vi "quiz 3.3.vi"() -> ()   [LabVIEW 2017]
panel:
  out "output string":string
  out "array":string[][](array[string])
  out "Tab Control":T1(tab)
  in  "Ingresar":bool
  in  "usuario":string
  in  "Contraseña":string
  in  "eliminar":bool
  in  "agregar":bool
  in  "TERMINAR":bool
  in  "Volver":bool
  in  "añadir":bool
  in  "contraseña":string
  in  "usuario":string
  in  "Quitar":bool
  in  "usuario a eliminar":string
  out "Seccion Inicada por:":string
  # "¿QUE DESEA REALIZAR?"
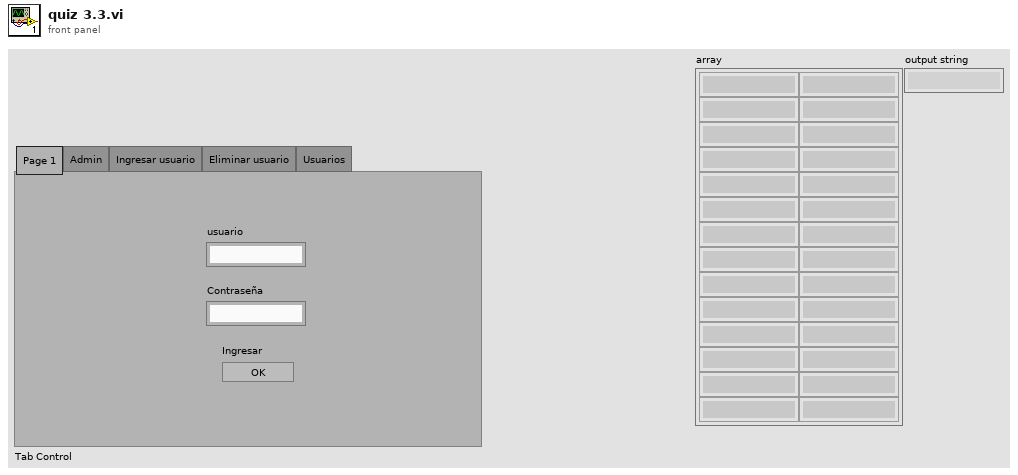
[diagram p1: front panel]
types:
  T1 = enum32{"Page 1", "Admin", "Ingresar usuario", "Eliminar usuario", "Usuarios"}
  T2 = enum16{"open", "replace", "create", "open or create", "replace or create", "replace or create with confirmation"}
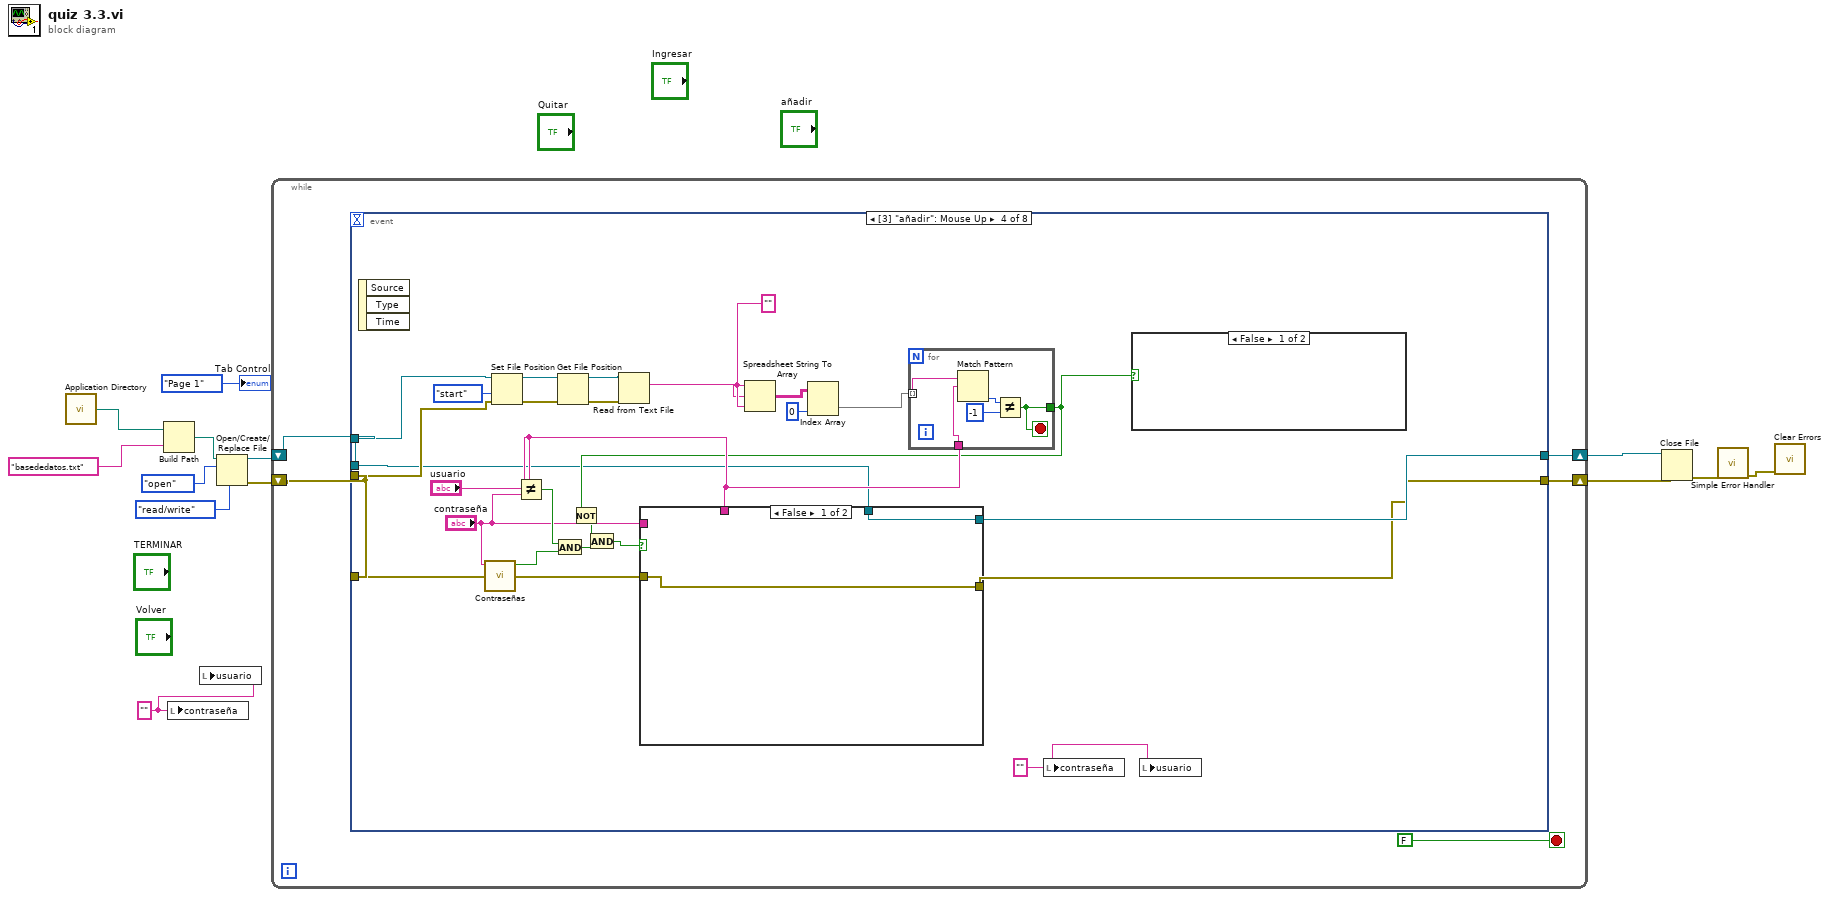
[diagram p0: block diagram]
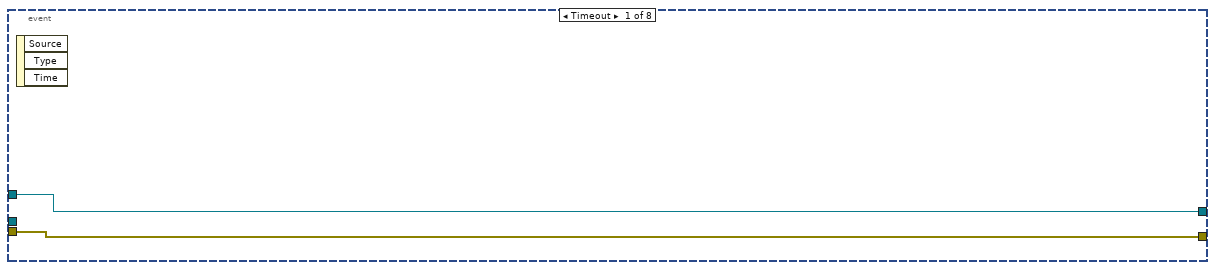
[diagram p2: hidden frame]
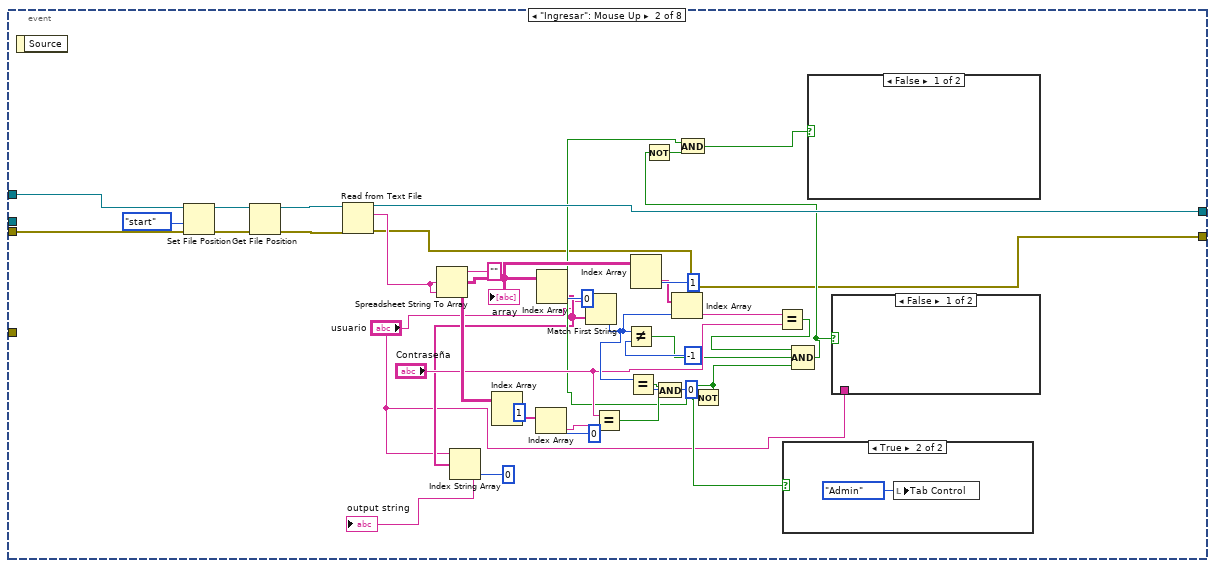
[diagram p3: hidden frame]
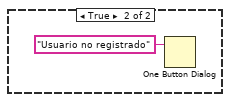
[diagram p4: hidden frame]
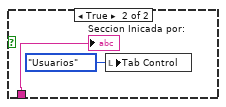
[diagram p5: hidden frame]
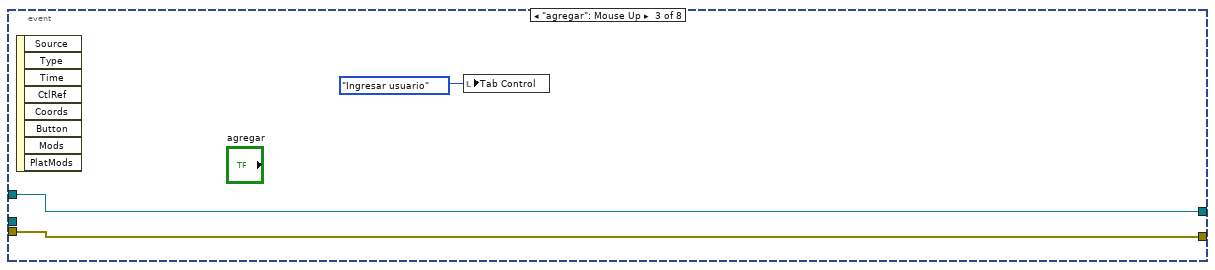
[diagram p7: hidden frame]
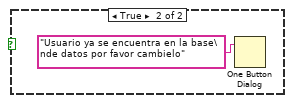
[diagram p8: hidden frame]
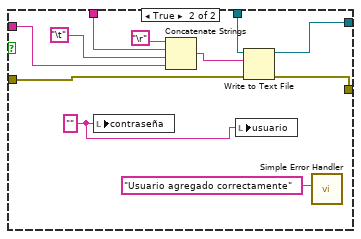
[diagram p9: hidden frame]
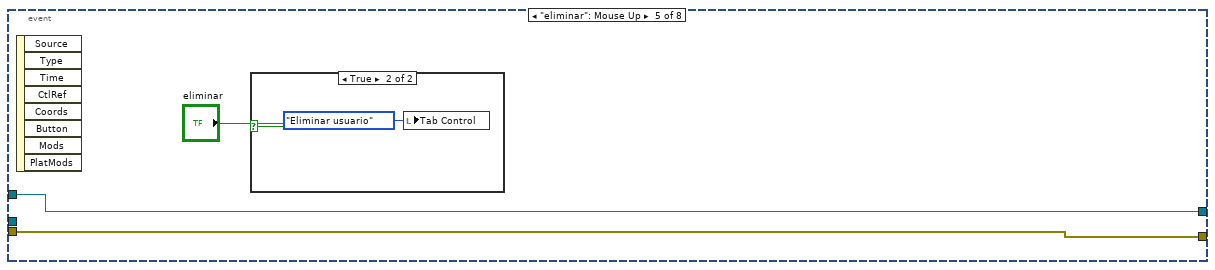
[diagram p10: hidden frame]
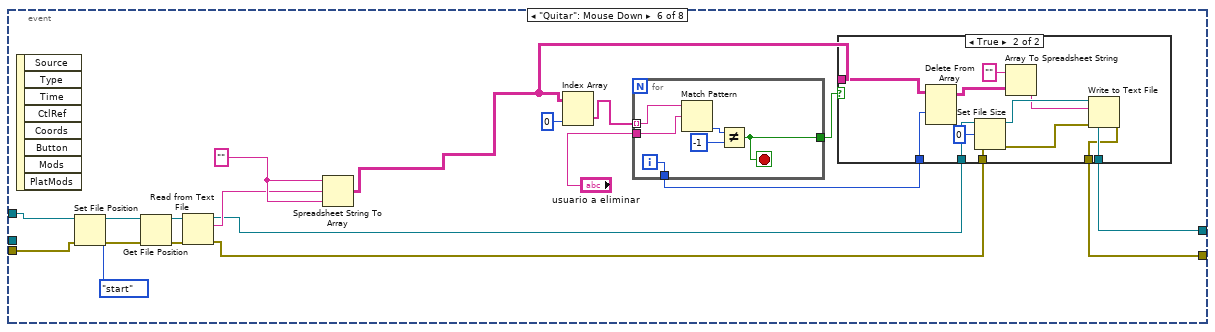
[diagram p12: hidden frame]
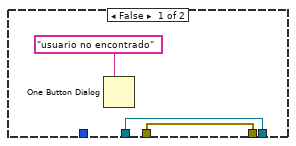
[diagram p13: hidden frame]
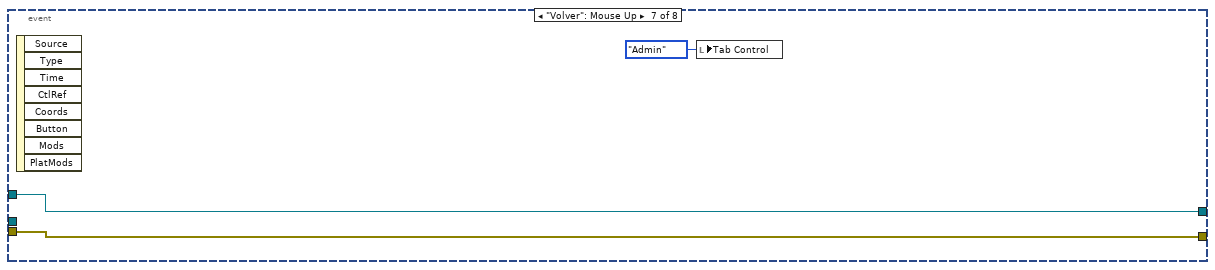
[diagram p14: hidden frame]
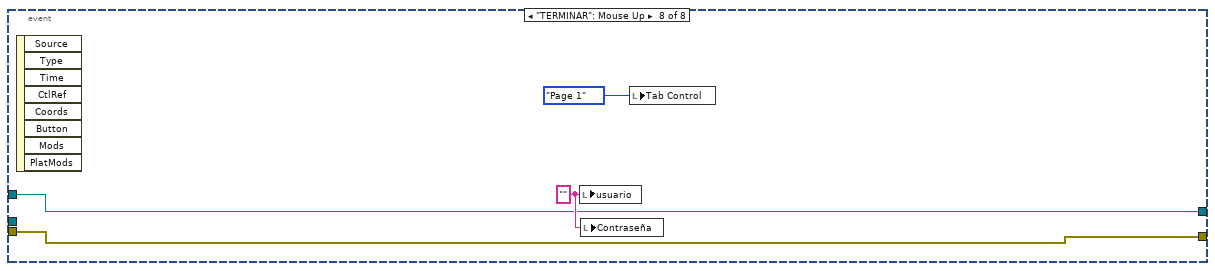
[diagram p15: hidden frame]
diagram:
  w1 = "" ("contraseña")
  n1 = call <vilib>:"Application Directory.vi"() -> ("Application Directory"=w10:path)
  n2 = Build Path(base path=w10, name or relative path="basededatos.txt") -> (appended path=w7:path)
  n3 = local write "contraseña"(w1) -> ()
  n4 = local write "usuario"(w1) -> ()
  n5 = Open/Create/Replace File(file path (use dialog)=w7, operation (0:open)=T2."open", access (0:read/write)=enum16{"read/write", "read-only", "write-only"}."read/write") -> (refnum out=w8:refnum<file>, error out=w5:errorcluster)  [unwired: 3 in, 1 out]
  n6 = while {
    shift-right: [w15] -> w11
    shift-left: w8 -> [w14]
    shift-right: [w16] -> w6
    shift-left: w5 -> [w17]
    stop <- FALSE stop-if-true
    n7 = event shown="[3] \"añadir\": Mouse Up" {
      selector: _ -> [_ _ _ _ _ _ _ _]
      dyn-events: _ -> [_ _ _ _ _ _ _ _]
      timeout: _ -> [_ _ _ _ _ _ _ _]
      tunnel: w14 -> [w20 w53 w64 w67 w109 w121 w154 w157]
      tunnel: [w20 w52 w64 w86 w109 w114 w154 w157] -> w15
      tunnel: w17 -> [w19 w48 w62 w82 w110 w120 w153 w156]
      tunnel: w17 -> [_ _ _ w88 _ _ _ _]
      tunnel: [w19 w22 w62 w69 w110 w113 w153 w156] -> w16
      tunnel: w14 -> [_ _ _ w66 _ _ _ _]
      event Timeout {
        n8 = event-data() -> ()  [unwired: 1 in, 3 out]
      }
      event "Ingresar": Mouse Up {
        n9 = event-data() -> ()  [unwired: 1 in, 1 out]
        n10 = Set File Position(refnum=w53, from (0:start)=enum16{"start", "end", "current"}."start", error in=w48) -> (refnum out=w57:refnum<file>, error out=w55:errorcluster)  [unwired: 1 in]
        n11 = Get File Position(4:w55, 7:w57) -> (0:w54:errorcluster, 3:w56:refnum<file>)  [unwired: 1 out]
        n12 = Read from Text File(file (use dialog)=w56, error in=w54) -> (refnum out=w52:refnum<file>, text=w50:string, error out=w22:errorcluster)  [unwired: 2 in, 1 out]
        n13 = Spreadsheet String To Array(format string="", spreadsheet string=w50, array type (2D Dbl)=w50) -> (array=w37:string[][])  [unwired: 1 in]
        "array" <- w37
        n14 = Index Array(array=w37, index (col)=1 ("disabled index (col)")) -> (element=w42:string[])  [unwired: 1 in]
        n15 = Index Array(array=w42, index=0) -> (element=w40:string)
        n16 = Index Array(array=w37, index (col)=0 ("disabled index (col)")) -> (element=w25:string[])  [unwired: 1 in]
        n17 = Index String Array(1:0 ("index"), 2:w25, 3:"usuario") -> (0:→"output string":string)
        n18 = Match First String(2:w25, 3:"usuario") -> (0:w34:i32)  [unwired: 1 out]
        n19 = Equal?(x="Contraseña", y=w40) -> (x = y?=w39:bool)
        n20 = Not Equal?(x=w34, y=-1) -> (x != y?=w30:bool)
        n21 = Equal?(x=w34, y=0) -> (x = y?=w44:bool)
        n22 = Index Array(array=w37, index (col)=1 ("disabled index (col)")) -> (element=w35:string[])  [unwired: 1 in]
        n23 = And(x=w44, y=w39) -> (x .and. y?=w38:bool)
        n24 = Index Array(array=w35, index=w34) -> (element=w33:string)
        n25 = Not(x=w38) -> (.not. x?=w26:bool)
        n26 = Equal?(x=w33, y="Contraseña") -> (x = y?=w31:bool)
        n27 = case shown="True" w38 {
          frame False {
          }
          frame True {
            n28 = local write "Tab Control"(T1."Admin" ("Tab Control")) -> ()
          }
        }
        n29 = Compound Arithmetic op=AND(w31, w30, w26) -> (w28:bool)
        n30 = Not(x=w28) -> (.not. x?=w29:bool)
        n31 = And(x=w26, y=w29) -> (x .and. y?=w27:bool)
        n32 = case shown="False" w27 {
          frame False {
          }
          frame True {
            n33 = One Button Dialog(message="Usuario no registrado") -> ()  [unwired: 1 in, 1 out]
          }
        }
        n34 = case shown="False" w28 {
          tunnel: "usuario" -> [_ w59]
          frame False {
          }
          frame True {
            n35 = local write "Tab Control"(T1."Usuarios" ("Tab Control")) -> ()
            "Seccion Inicada por:" <- w59
          }
        }
      }
      event "agregar": Mouse Up {
        n36 = event-data() -> ()  [unwired: 1 in, 8 out]
        n37 = local write "Tab Control"(T1."Ingresar usuario" ("Tab Control")) -> ()
      }
      event "añadir": Mouse Up {
        w68 = "" ("contraseña")
        w79 = "" ("format string")
        n38 = event-data() -> ()  [unwired: 1 in, 3 out]
        n39 = call "Contraseñas.vi"("String"="contraseña") -> ("Contraseña Correcta?"=w65:bool)  [unwired: 10 in]
        n40 = Set File Position(refnum=w67, from (0:start)=enum16{"start", "end", "current"}."start", error in=w82) -> (refnum out=w85:refnum<file>, error out=w81:errorcluster)  [unwired: 1 in]
        n41 = Not Equal?(x="usuario", y="contraseña") -> (x != y?=w89:bool)
        n42 = And(x=w89, y=w65) -> (x .and. y?=w73:bool)
        n43 = Get File Position(4:w81, 7:w85) -> (0:w80:errorcluster, 3:w84:refnum<file>)  [unwired: 1 out]
        n44 = Read from Text File(file (use dialog)=w84, error in=w80) -> (text=w78:string)  [unwired: 2 in, 3 out]
        n45 = Spreadsheet String To Array(format string=w79, spreadsheet string=w78, array type (2D Dbl)=w79) -> (array=w77:string[][])  [unwired: 1 in]
        n46 = Index Array(array=w77, index (col)=0 ("disabled index (col)")) -> (element=w75:string[])  [unwired: 1 in]
        n47 = for {
          tunnel: w75 -> [w95] mode=indexing
          tunnel: "usuario" -> [w94]
          tunnel: [w91] -> w71
          stop <- w91 stop-if-true
          n48 = Match Pattern(string=w95, regular expression=w94) -> (offset past match=w93:i32)  [unwired: 1 in, 3 out]
          n49 = Not Equal?(x=w93, y=-1) -> (x != y?=w91:bool)
        }
        n50 = Not(x=w71) -> (.not. x?=w70:bool)
        n51 = And(x=w70, y=w73) -> (x .and. y?=w72:bool)
        n52 = case shown="False" w72 {
          tunnel: w88 -> [w97 w108]
          tunnel: w66 -> [w96 w107]
          tunnel: [w97 w106] -> w69
          tunnel: [w96 w105] -> w86
          tunnel: "usuario" -> [_ w104]
          tunnel: "contraseña" -> [_ w103]
          frame False {
          }
          frame True {
            w98 = "" ("contraseña")
            n53 = local write "contraseña"(w98) -> ()
            n54 = Concatenate Strings("\r", w104, "\t", w103) -> (w102:string)
            n55 = local write "usuario"(w98) -> ()
            n56 = Write to Text File(file (use dialog)=w107, text=w102, error in=w108) -> (refnum out=w105:refnum<file>, error out=w106:errorcluster)  [unwired: 1 in, 1 out]
            n57 = call <vilib>:"Simple Error Handler.vi"("error source (\" \")"="Usuario agregado correctamente" ("error source (\" \")")) -> ()  [unwired: 4 in, 5 out]
          }
        }
        n58 = local write "contraseña"(w68) -> ()
        n59 = case shown="False" w71 {
          frame False {
          }
          frame True {
            n60 = One Button Dialog(message="Usuario ya se encuentra en la base\nde datos por favor cambielo") -> ()  [unwired: 1 in, 1 out]
          }
        }
        n61 = local write "usuario"(w68) -> ()
      }
      event "eliminar": Mouse Up {
        n62 = event-data() -> ()  [unwired: 1 in, 8 out]
        n63 = case shown="True" "eliminar" {
          frame False {
          }
          frame True {
            n64 = local write "Tab Control"(T1."Eliminar usuario" ("Tab Control")) -> ()
          }
        }
      }
      event "Quitar": Mouse Down {
        w131 = "" ("format string")
        n65 = event-data() -> ()  [unwired: 1 in, 8 out]
        n66 = Set File Position(refnum=w121, from (0:start)=enum16{"start", "end", "current"}."start", error in=w120) -> (refnum out=w123:refnum<file>, error out=w119:errorcluster)  [unwired: 1 in]
        n67 = Get File Position(4:w119, 7:w123) -> (0:w118:errorcluster, 3:w117:refnum<file>)  [unwired: 1 out]
        n68 = Read from Text File(file (use dialog)=w117, error in=w118) -> (refnum out=w116:refnum<file>, text=w130:string, error out=w115:errorcluster)  [unwired: 2 in, 1 out]
        n69 = Spreadsheet String To Array(format string=w131, spreadsheet string=w130, array type (2D Dbl)=w131) -> (array=w125:string[][])  [unwired: 1 in]
        n70 = Index Array(array=w125, index (col)=0 ("disabled index (col)")) -> (element=w127:string[])  [unwired: 1 in]
        n71 = for {
          tunnel: w127 -> [w148] mode=indexing
          tunnel: [w150] -> w126
          tunnel: "usuario a eliminar" -> [w149]
          tunnel: [w147] -> w124
          i -> [w147]
          stop <- w150 stop-if-true
          n72 = Match Pattern(string=w148, regular expression=w149) -> (offset past match=w152:i32)  [unwired: 1 in, 3 out]
          n73 = Not Equal?(x=w152, y=-1) -> (x != y?=w150:bool)
        }
        n74 = case shown="True" w126 {
          tunnel: w125 -> [_ w146]
          tunnel: w124 -> [_ w145]
          tunnel: w116 -> [w132 w144]
          tunnel: w115 -> [w133 w143]
          tunnel: [w132 w138] -> w114
          tunnel: [w133 w137] -> w113
          frame False {
            n75 = One Button Dialog(message="usuario no encontrado") -> ()  [unwired: 1 in, 1 out]
          }
          frame True {
            n76 = Delete From Array(array=w146, index (row)=w145) -> (array with subset deleted=w136:string[][])  [unwired: 2 in, 1 out]
            n77 = Set File Size(4:w143, 6:i64 0 ("offset (in bytes) (0)"), 7:w144) -> (0:w139:errorcluster, 3:w142:refnum<file>)
            n78 = Array To Spreadsheet String(array=w136, 3:"" ("format string")) -> (spreadsheet string=w140:string)  [unwired: 1 in]
            n79 = Write to Text File(file (use dialog)=w142, text=w140, error in=w139) -> (refnum out=w138:refnum<file>, error out=w137:errorcluster)  [unwired: 1 in, 1 out]
          }
        }
      }
      event "Volver": Mouse Up {
        n80 = event-data() -> ()  [unwired: 1 in, 8 out]
        n81 = local write "Tab Control"(T1."Admin" ("Tab Control")) -> ()
      }
      event "TERMINAR": Mouse Up {
        w158 = "" ("usuario")
        n82 = event-data() -> ()  [unwired: 1 in, 8 out]
        n83 = local write "usuario"(w158) -> ()
        n84 = local write "Contraseña"(w158) -> ()
        n85 = local write "Tab Control"(T1."Page 1" ("Tab Control")) -> ()
      }
    }
  }
  n86 = Close File(refnum=w11, error in=w6) -> (error out=w4:errorcluster)  [unwired: 1 out]
  n87 = call <vilib>:"Simple Error Handler.vi"("error in (no error)"=w4) -> ("error out"=w3:errorcluster)  [unwired: 4 in, 4 out]
  n88 = call <vilib>:"Clear Errors.vi"("error in (no error)"=w3) -> ()  [unwired: 5 in, 2 out]
  "Tab Control" <- T1."Page 1" ("Tab Control")
